vi "Destroy.vi"(0 "reference in":refnum<class "TDMS.lvclass">, 5 "error in (no error)":errorcluster) -> (14 "reference out":refnum<class "TDMS.lvclass">, 19 "error out":errorcluster)   [LabVIEW 2022 SP3, in "TDMS.lvclass"]
doc: "Destructor."
uses:
  TDMS.lvclass
  API/Generic Utilities_class/Generic Utilities.lvclass
  API/GSwFormDSP_class/GSwFormDSP.lvclass
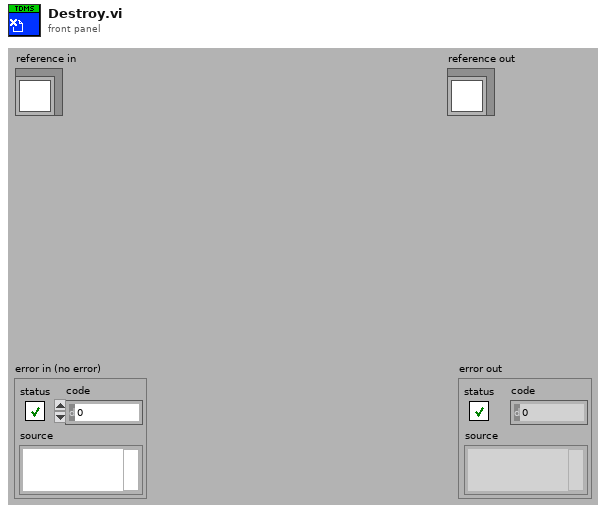
[diagram p1: front panel]
types:
  T1 = typedef "TDMS.lvclass/ObjectAttributes.ctl" = cluster{"Time Data":refnum<class "GSwFormDSP.lvclass">, "New Time Data Obj?":bool}
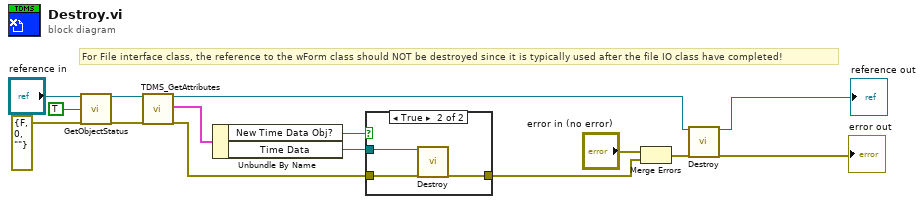
[diagram p0: block diagram]
diagram:
  # "For File interface class, the reference to the wForm class should NOT be destroyed since it is typically used after the file IO class have completed!"
  n1 = call-dynamic "GetObjectStatus.vi"("reference in"="reference in", "simple info (F)"=TRUE ("simple info"), "error in (no error)"=errorcluster {"status"=FALSE, "code"=0, "source"=""}) -> ("reference out"=w8:refnum<class "TDMS.lvclass">, "error out"=w6:errorcluster)  [unwired: 5 in, 10 out]
  n2 = call "TDMS_GetAttributes.vi"("reference in"=w8, "error in (no error)"=w6) -> ("reference out"=w7:refnum<class "TDMS.lvclass">, "attributes"=w5:T1, "error out"=w2:errorcluster)  [unwired: 14 in, 1 out]
  n3 = Unbundle By Name(w5) -> ("New Time Data Obj?"=w4:bool, "Time Data"=w3:refnum<class "GSwFormDSP.lvclass">)
  n4 = case shown="True" w4 {
    tunnel: w3 -> [_ w19]
    tunnel: w2 -> [w16 w18]
    tunnel: [w16 w17] -> w1
    frame False {
    }
    frame True {
      n5 = call-dynamic "Destroy.vi"("reference in"=w19, "error in (no error)"=w18) -> ("error out"=w17:errorcluster)  [unwired: 16 in, 1 out]
    }
  }
  n6 = Merge Errors("error in (no error)", w1) -> (w14:errorcluster)
  n7 = call-parent "Destroy.vi"("reference in"=w7, "error in (no error)"=w14) -> ("reference out"=→"reference out":refnum<class "TDMS.lvclass">, "error out"=→"error out":errorcluster)  [unwired: 16 in]
